vi "CreateStandardEvents.vi"(8 "error in":errorcluster) -> (0 "error out":errorcluster, 3 "standard events":T1)   [LabVIEW 2025, in "CEF.lvlib" / "CEF_Node.lvclass"]
doc: "Copyright 2017 National Instruments Corporation\n\nLicensed under the Apache License, Version 2.0 (the \"License\"); you may not use this file except in compliance with the License. You may obtain a copy of the License at http://www.apache.org/licenses/LICENSE-2.0\nUnless required by applicable law or agreed to in writing, software distributed under the License is distributed on an \"AS IS\" BASIS, WITHOUT WARRANTIES OR CONDITIONS OF ANY KIND, either express or implied. See the License for the specific language governing permissions and limitations under the License."
uses:
  CEF_Node.lvclass
  StandardEvents.ctl
  UserEventRef.ctl
  Controls/EventCluster.ctl
  NodeChangeEvent.ctl
  NodeRef.ctl
  CacheState.ctl
  RefreshUIEvent.ctl
  StopEvent.ctl
  CEF_Node.lvclass/CEF_Node.ctl
  CEF.lvlib
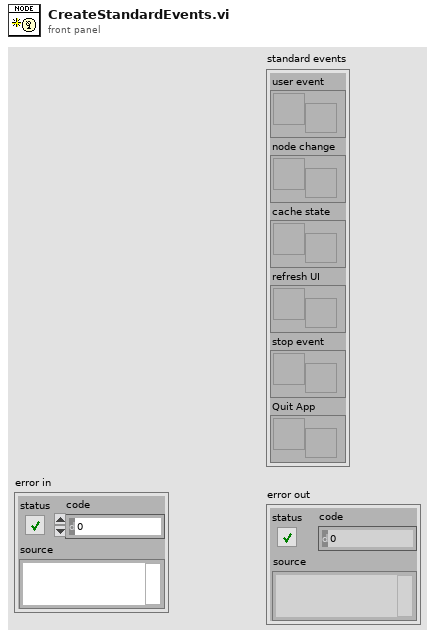
[diagram p1: front panel]
types:
  T1 = typedef "CEF.lvlib/CEF_Node.lvclass/StandardEvents.ctl" = cluster{"user event":T2, "node change":T3, "cache state":T4, "refresh UI":T5, "stop event":T6, "Quit App":refnum<user-event>}
  T2 = typedef "CEF.lvlib/CEF_Node.lvclass/UserEventRef.ctl" = refnum<user-event>
  T3 = typedef "CEF.lvlib/CEF_Node.lvclass/NodeChangeEvent.ctl" = refnum<user-event>
  T4 = typedef "CEF.lvlib/CEF_Node.lvclass/CacheState.ctl" = refnum<user-event>
  T5 = typedef "CEF.lvlib/CEF_Node.lvclass/RefreshUIEvent.ctl" = refnum<user-event>
  T6 = typedef "CEF.lvlib/CEF_Node.lvclass/StopEvent.ctl" = refnum<user-event>
  T7 = typedef "CEF.lvlib/CEF_Node.lvclass/NodeRef.ctl" = refnum<data-value>
  T8 = typedef "CEF.lvlib/EventCluster.ctl" = cluster{"command":string, "data":string}
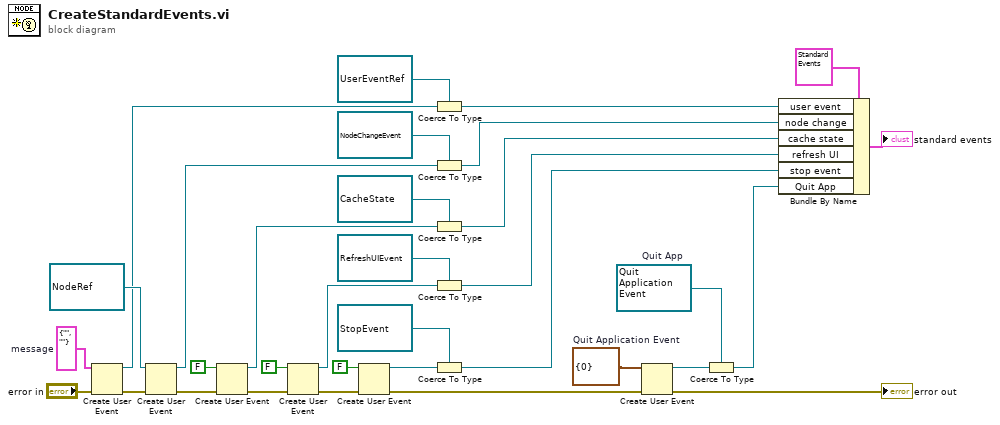
[diagram p0: block diagram]
diagram:
  w2 = refnum<user-event> refnum  # Quit App
  w4 = cluster{"Number":i32} {"Number"=0}  # Quit Application Event
  w26 = T8 {"command"="", "data"=""}  # message
  n1 = Create User Event(user event datatype=w26, error in="error in") -> (user event=w21:refnum<user-event>, error out=w30:errorcluster)
  n2 = Create User Event(user event datatype=T7 refnum ("node ref"), error in=w30) -> (user event=w17:refnum<user-event>, error out=w29:errorcluster)
  n3 = Create User Event(user event datatype=FALSE ("cache state"), error in=w29) -> (user event=w18:refnum<user-event>, error out=w28:errorcluster)
  n4 = Create User Event(user event datatype=FALSE ("refresh UI"), error in=w28) -> (user event=w19:refnum<user-event>, error out=w27:errorcluster)
  n5 = Create User Event(user event datatype=FALSE ("stop"), error in=w27) -> (user event=w20:refnum<user-event>, error out=w6:errorcluster)
  n6 = Coerce To Type(0:w21, 1:T2 refnum ("user event")) -> (2:w16:T2)
  n7 = Coerce To Type(0:w17, 1:T3 refnum ("node change")) -> (2:w15:T3)
  n8 = Coerce To Type(0:w18, 1:T4 refnum ("cache state")) -> (2:w14:T4)
  n9 = Coerce To Type(0:w19, 1:T5 refnum ("refresh UI")) -> (2:w13:T5)
  n10 = Coerce To Type(0:w20, 1:T6 refnum ("stop event")) -> (2:w12:T6)
  n11 = Create User Event(user event datatype=w4, error in=w6) -> (user event=w3:refnum<user-event>, error out=→"error out":errorcluster)
  n12 = Coerce To Type(0:w3, 1:w2) -> (2:w1:refnum<user-event>)
  n13 = Bundle By Name(cluster=T1 {"user event"=refnum, "node change"=refnum, "cache state"=refnum, "refresh UI"=refnum, "stop event"=refnum, "Quit App"=refnum} ("standard events"), "user event"=w16, "node change"=w15, "cache state"=w14, "refresh UI"=w13, "stop event"=w12, "Quit App"=w1) -> (→"standard events":T1)
